vi "MinDisplac(FinishP)1.vi"(4 "error IN":errorcluster, 7 "[IN] (X,Y,dX,dY)":dbl[][](array[numeric])) -> (0 "error OUT":errorcluster, 3 "[OUT] (X,Y,dX,dY)":dbl[][](array[numeric]))   [LabVIEW 2013]
doc: "If the destination point in displacements are the same, subprogram saves only with minimal displacements between found variants"
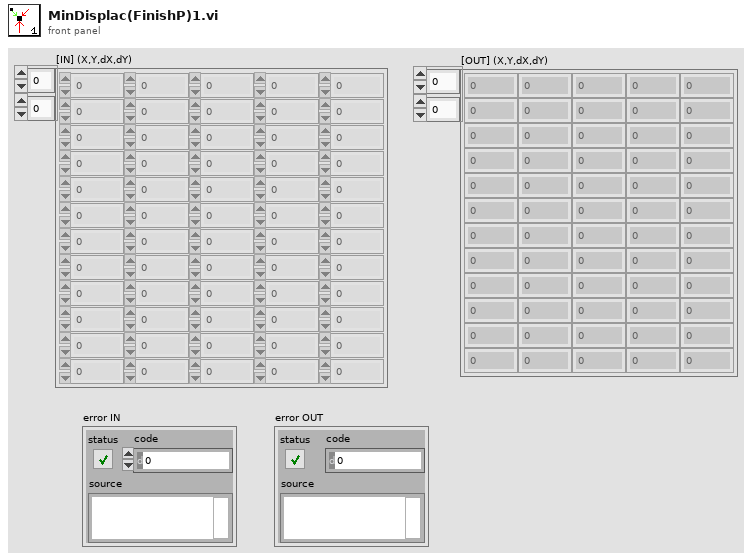
[diagram p1: front panel]
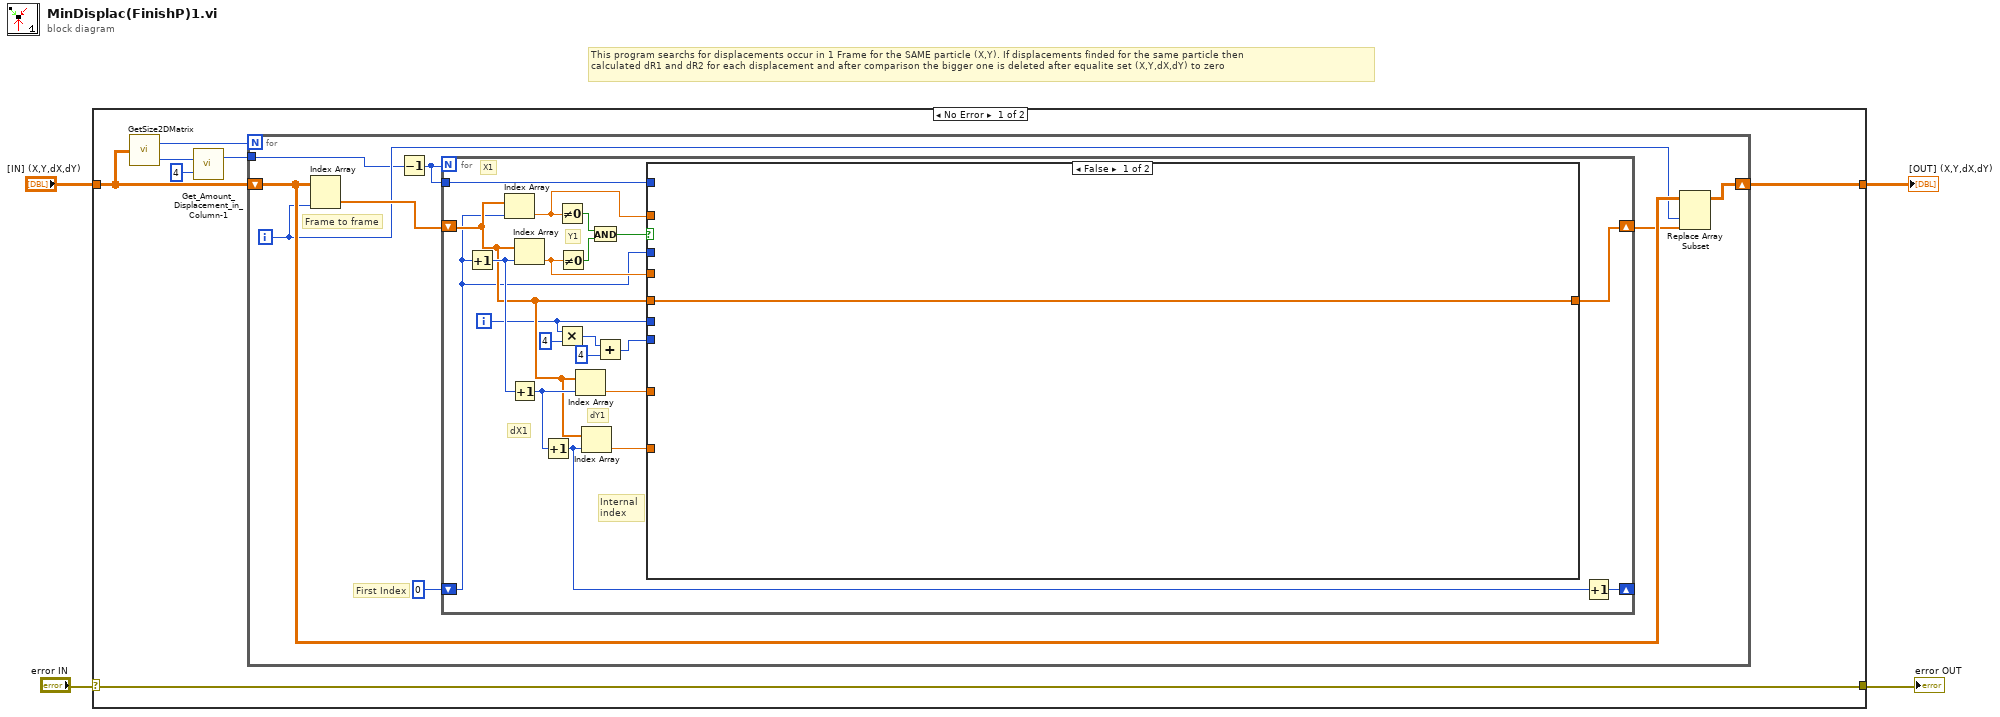
[diagram p0: block diagram]
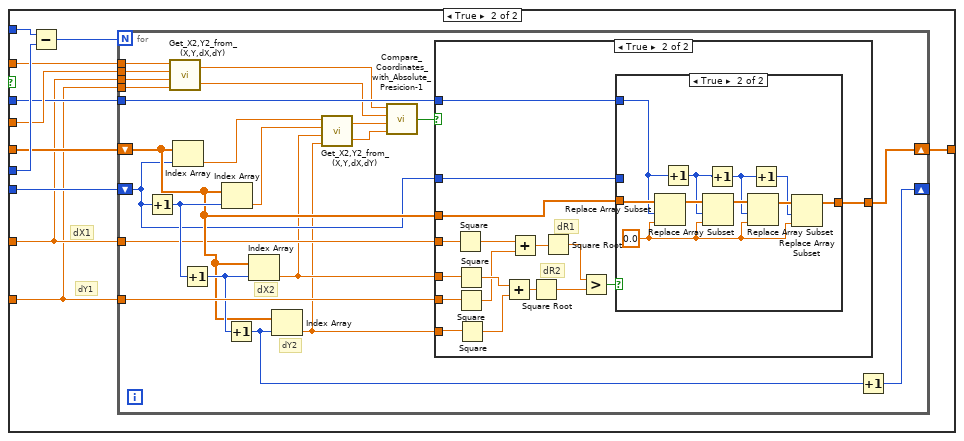
[diagram p2: hidden frame]
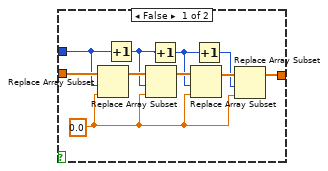
[diagram p4: hidden frame]
diagram:
  # "This program searchs for displacements occur in 1 Frame for the SAME particle (X,Y). If displacements finded for the same particle then \ncalculated dR1 and dR2 for each displacement and after comparison the bigger one is deleted after equalite set (X,Y,dX,dY) to zero"
  n1 = case shown="No Error" "error IN" {
    selector: "error IN" -> [w8 w114]
    tunnel: [w11 w113] -> w4
    tunnel: "[IN] (X,Y,dX,dY)" -> [w10 w113]
    tunnel: [w8 w114] -> w1
    frame No Error {
      n2 = call "GetSize2DMatrix.vi"("Array IN (2D)"=w10) -> ("# Cols"=w9:i32, "# Rows"=w7:i32)
      n3 = call "Get_Amount_Displacement_in_Column-1.vi"("multiplier"=4, "# Rows"=w7) -> ("Displ amount"=w6:i32)  [unwired: 1 out]
      n4 = for {
        N: w9 -> [_]
        shift-right: [w13] -> w11
        shift-left: w10 -> [w16]
        tunnel: w6 -> [w12]
        i -> [w15]
        # "First Index"
        # "Frame to frame"
        n5 = Index Array(array=w16, index (col)=w15) -> (element=w19:dbl[])  [unwired: 1 in]
        n6 = Decrement(x=w12) -> (x-1=w17:i32)
        n7 = for {
          N: w17 -> [_]
          shift-right: [w20] -> w14
          shift-left: w19 -> [w31]
          shift-right: [w29] -> _
          shift-left: 0 -> [w21]
          tunnel: w17 -> [w36]
          i -> [w26]
          # "dX1"
          # "dY1"
          # "Internal \nindex"
          # "Y1"
          # "X1"
          n8 = Increment(x=w21) -> (x+1=w33:i32)
          n9 = Index Array(array=w31, index=w21) -> (element=w35:dbl)
          n10 = Increment(x=w33) -> (x+1=w32:i32)
          n11 = Index Array(array=w31, index=w33) -> (element=w34:dbl)
          n12 = Increment(x=w32) -> (x+1=w30:i32)
          n13 = Not Equal To 0?(x=w35) -> (x != 0?=w39:bool)
          n14 = Multiply(x=w26, y=4) -> (x*y=w24:i32)
          n15 = Not Equal To 0?(x=w34) -> (x != 0?=w38:bool)
          n16 = Index Array(array=w31, index=w32) -> (element=w28:dbl)
          n17 = Index Array(array=w31, index=w30) -> (element=w27:dbl)
          n18 = And(x=w39, y=w38) -> (x .and. y?=w37:bool)
          n19 = Add(x=w24, y=4) -> (x+y=w23:i32)
          n20 = case shown="False" w37 {
            tunnel: w36 -> [_ w51]
            tunnel: w26 -> [_ w50]
            tunnel: w35 -> [_ w47]
            tunnel: w34 -> [_ w46]
            tunnel: w31 -> [w40 w48]
            tunnel: [w40 w45] -> w20
            tunnel: w28 -> [_ w42]
            tunnel: w27 -> [_ w41]
            tunnel: w23 -> [_ w44]
            tunnel: w21 -> [_ w43]
            frame False {
            }
            frame True {
              # "dX1"
              # "dY1"
              n21 = Subtract(x=w51, y=w50) -> (x-y=w49:i32)
              n22 = for {
                N: w49 -> [_]
                shift-right: [w67] -> w45
                shift-left: w48 -> [w69]
                tunnel: w47 -> [w63]
                tunnel: w46 -> [w62]
                shift-right: [w70] -> _
                shift-left: w44 -> [w66]
                tunnel: w42 -> [w65]
                tunnel: w41 -> [w74]
                tunnel: w43 -> [w68]
                tunnel: w42 -> [w61]
                tunnel: w41 -> [w60]
                # "dY2"
                # "dX2"
                n23 = Increment(x=w66) -> (x+1=w73:i32)
                n24 = call "Get_X2,Y2_from_(X,Y,dX,dY).vi"("dY"=w60, "dX"=w61, "Y1"=w62, "X1"=w63) -> ("Y2 = (Y1+dY)"=w58:dbl, "X2 = (X1+dX)"=w59:dbl)
                n25 = Index Array(array=w69, index=w66) -> (element=w57:dbl)
                n26 = Increment(x=w73) -> (x+1=w72:i32)
                n27 = Index Array(array=w69, index=w73) -> (element=w56:dbl)
                n28 = Increment(x=w72) -> (x+1=w71:i32)
                n29 = Index Array(array=w69, index=w72) -> (element=w55:dbl)
                n30 = Index Array(array=w69, index=w71) -> (element=w54:dbl)
                n31 = call "Get_X2,Y2_from_(X,Y,dX,dY).vi"("dY"=w54, "dX"=w55, "Y1"=w56, "X1"=w57) -> ("Y2 = (Y1+dY)"=w52:dbl, "X2 = (X1+dX)"=w53:dbl)
                n32 = call "Compare_Coordinates_with_Absolute_Presicion-1.vi"("X 1"=w59, "Y 1"=w58, "X 2"=w53, "Y 2"=w52) -> ("[OUT] Same coordinates?"=w64:bool)  [unwired: 1 in]
                n33 = case shown="True" w64 {
                  tunnel: w65 -> [_ w92]
                  tunnel: w74 -> [_ w90]
                  tunnel: w54 -> [_ w89]
                  tunnel: w55 -> [_ w91]
                  tunnel: w69 -> [w75 w81]
                  tunnel: w68 -> [_ w80]
                  tunnel: [w75 w79] -> w67
                  tunnel: w66 -> [_ w78]
                  frame False {
                  }
                  frame True {
                    # "dR2"
                    # "dR1"
                    n34 = Square(x=w92) -> (x^2=w86:dbl)
                    n35 = Square(x=w91) -> (x^2=w88:dbl)
                    n36 = Square(x=w90) -> (x^2=w77:dbl)
                    n37 = Square(x=w89) -> (x^2=w76:dbl)
                    n38 = Add(x=w88, y=w76) -> (x+y=w87:dbl)
                    n39 = Add(x=w86, y=w77) -> (x+y=w85:dbl)
                    n40 = Square Root(x=w87) -> (sqrt(x)=w83:dbl)
                    n41 = Square Root(x=w85) -> (sqrt(x)=w84:dbl)
                    n42 = Greater?(x=w84, y=w83) -> (0:w82:bool)
                    n43 = case shown="True" w82 {
                      tunnel: w81 -> [w95 w112]
                      tunnel: w80 -> [_ w110]
                      tunnel: [w93 w103] -> w79
                      tunnel: w78 -> [w94 _]
                      frame False {
                        w99 = 0.0 ("new element/subarray")
                        n44 = Replace Array Subset(array=w95, new element=w99, index=w94) -> (w102:dbl[])
                        n45 = Increment(x=w94) -> (x+1=w98:i32)
                        n46 = Replace Array Subset(array=w102, new element=w99, index=w98) -> (w101:dbl[])
                        n47 = Increment(x=w98) -> (x+1=w97:i32)
                        n48 = Replace Array Subset(array=w101, new element=w99, index=w97) -> (w100:dbl[])
                        n49 = Increment(x=w97) -> (x+1=w96:i32)
                        n50 = Replace Array Subset(array=w100, new element=w99, index=w96) -> (w93:dbl[])
                      }
                      frame True {
                        w107 = 0.0 ("new element/subarray")
                        n51 = Replace Array Subset(array=w112, new element=w107, index=w110) -> (w111:dbl[])
                        n52 = Increment(x=w110) -> (x+1=w106:i32)
                        n53 = Replace Array Subset(array=w111, new element=w107, index=w106) -> (w109:dbl[])
                        n54 = Increment(x=w106) -> (x+1=w105:i32)
                        n55 = Replace Array Subset(array=w109, new element=w107, index=w105) -> (w108:dbl[])
                        n56 = Increment(x=w105) -> (x+1=w104:i32)
                        n57 = Replace Array Subset(array=w108, new element=w107, index=w104) -> (w103:dbl[])
                      }
                    }
                  }
                }
                n58 = Increment(x=w71) -> (x+1=w70:i32)
              }
            }
          }
          n59 = Increment(x=w30) -> (x+1=w29:i32)
        }
        n60 = Replace Array Subset(array=w16, new element=w14, index (col)=w15) -> (w13:dbl[][])  [unwired: 1 in]
      }
    }
    frame Error {
    }
  }
  "error OUT" <- w1
  "[OUT] (X,Y,dX,dY)" <- w4
